vi "test_sum_aux.vi"(2 "Z mismatch":waveform(sgl)[](array[waveform]), 3 "Sum amplitudes":sgl[][](array[numeric])) -> (0 "Real 2D Array":sgl[][](array[numeric]), 1 "Array":sgl[][](array[numeric]))   [LabVIEW 2011]
uses:
  <vilib>/Analysis/Matrix/Numeric/Conversions/Array To Matrix - RA.vi
  <vilib>/Analysis/Matrix/Numeric/Conversions/Matrix To Array - RM.vi
  <vilib>/Waveform/WDTOps.llb/WDT Get XY Value DBL.vi
  <vilib>/Analysis/Matrix/NI_Matrix.lvlib
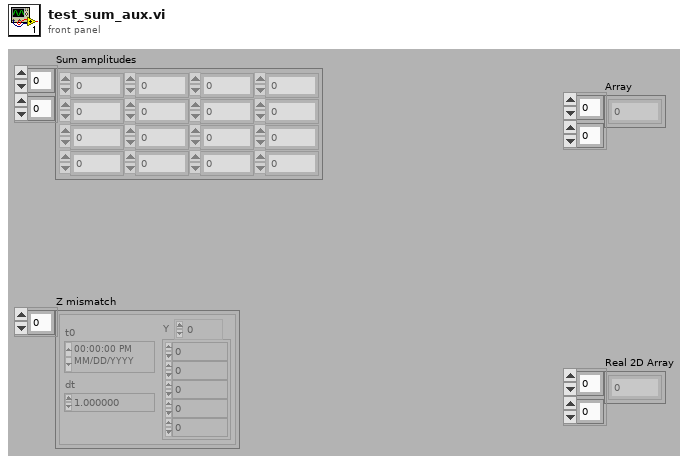
[diagram p1: front panel]
types:
  T1 = typedef "NI_Matrix.lvlib/RealMatrix.ctl" = dbl[][]
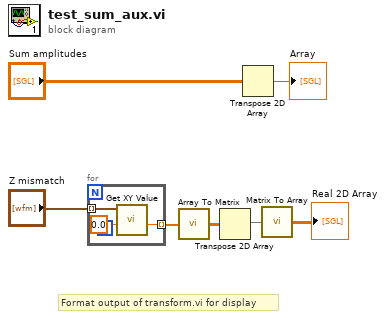
[diagram p0: block diagram]
diagram:
  # "Format output of transform.vi for display"
  n1 = for {
    tunnel: "Z mismatch" -> [w10] mode=indexing
    tunnel: [w8] -> w4 mode=indexing
    n2 = call-poly <vilib>:"Get XY Value.vi"("Y position"=0.0, "waveform in"=w10) -> ("Y value"=w8:dbl)  [unwired: 2 in, 7 out]
  }
  n3 = call-poly <vilib>:"Array To Matrix.vi"("Real 1D Array"=w4) -> ("Real Matrix (Column Vector)"=w5:T1)
  n4 = Transpose 2D Array(2D array=w5) -> (transposed array=w6:T1)
  n5 = Transpose 2D Array(2D array="Sum amplitudes") -> (transposed array=→"Array":sgl[][])
  n6 = call-poly <vilib>:"Matrix To Array.vi"("Real Matrix"=w6) -> ("Real 2D Array"=→"Real 2D Array":dbl[][])
